vi "Inverse Kinematics Test.vi"() -> ()   [LabVIEW 2023]
uses:
  <vilib>/Analysis/coordinate.llb/Angle Units.ctl
  <vilib>/Analysis/coordinate.llb/Wrap Angle (scalar).vi
  <vilib>/Analysis/NI_AAL_Angle.lvlib
panel:
  in  "Turning Rate":dbl
  in  "Pod Max Turn Rate":dbl
  in  "stop":bool
  in  "Hide Components?":bool
  in  "dt":dbl
  in  "# Points":i32
  out "Expected Trajectory":cluster{dbl[], dbl[]}(graph)
  in  "Angular Velocity":dbl(slide) scale=-180.0..180.0
  out "Arcade Inputs":picture
  out "Visualization":cluster{dbl[], dbl[]}[](graph)
  in  "Radii":T1={"LF"=[-2.0, 2.0], "LB"=[-2.0, -2.0], "RF"=[2.0, 2.0], "RB"=[2.0, -2.0]} {"RB" format="%.2f"; "RF" format="%.2f"; "LB" format="%.2f"; "LF" format="%.2f"}
  # "Front (1)"
  # "Left (-1)"
  # "Right (1)"
  # "Back (-1)"
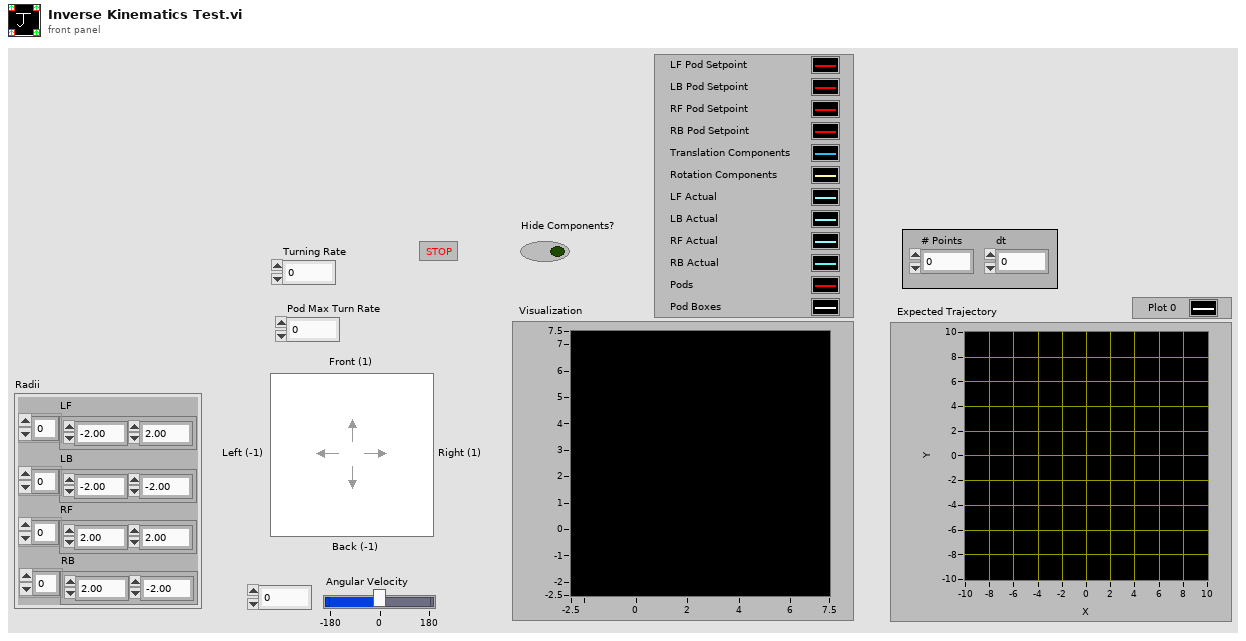
[diagram p1: front panel]
types:
  T1 = cluster{"LF":dbl[], "LB":dbl[], "RF":dbl[], "RB":dbl[]}
  T2 = cluster{"Plot.Plot Color":u32, "Plot.Line Style":u8}
  T3 = typedef "LVMouseTypeDef.ctl" = cluster{"Mouse Position":cluster{"X":i32, "Y":i32}, "Mouse Modifiers":cluster{"Button Down":bool, "Shift Mod":bool, "Menu Mod":bool, "Option Mod":bool}}
  T4 = typedef "LVBoundsTypeDef.ctl" = cluster{"Width":u32, "Height":u32}
  T5 = typedef "Pod Setpoints.ctl" = cluster{"Left Front":cluster{"Velocity":dbl, "Theta":dbl}, "Left Back":cluster{"Velocity":dbl, "Theta":dbl}, "Right Front":cluster{"Velocity":dbl, "Theta":dbl}, "Right Back":cluster{"Velocity":dbl, "Theta":dbl}}
  T6 = typedef "NI_AAL_Angle.lvlib/Angle Units.ctl" = i32
  T7 = cluster{"[0]":dbl, "[1]":dbl, "[2]":dbl, "[3]":dbl}
  T8 = cluster{"[0]":cluster{"Velocity":dbl, "Theta":dbl}, "[1]":cluster{"Velocity":dbl, "Theta":dbl}, "[2]":cluster{"Velocity":dbl, "Theta":dbl}, "[3]":cluster{"Velocity":dbl, "Theta":dbl}}
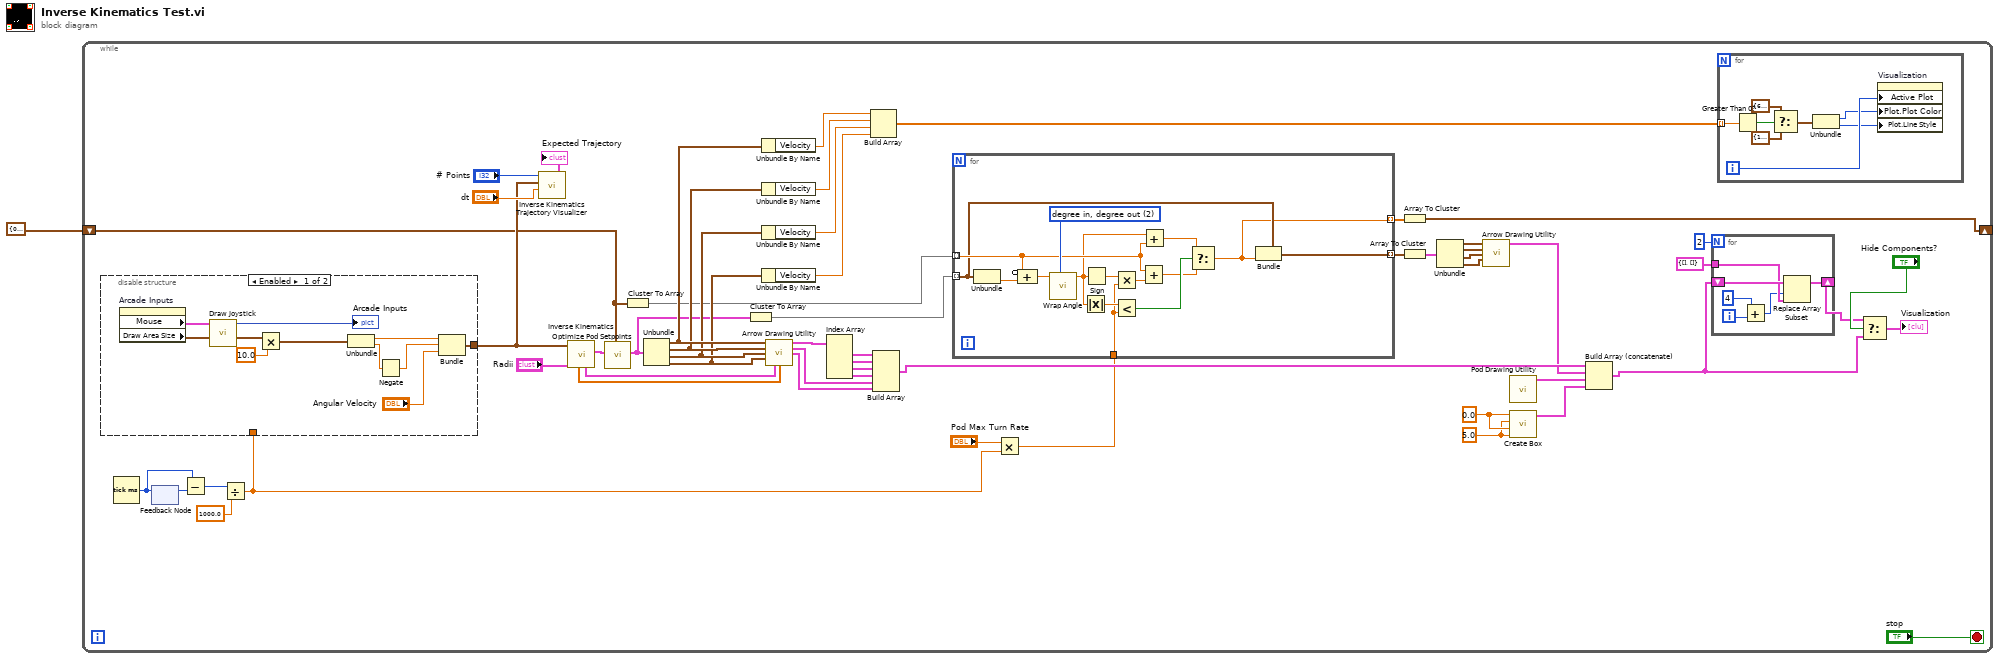
[diagram p0: block diagram]
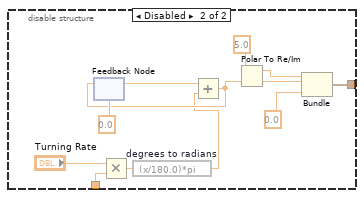
[diagram p2: hidden frame]
diagram:
  n1 = while {
    shift-right: [w20] -> _
    shift-left: cluster{"LF":dbl, "LB":dbl, "RF":dbl, "RB":dbl} {"LF"=0.0, "LB"=0.0, "RF"=0.0, "RB"=0.0} ("Current Pod Steering") -> [w25]
    stop <- "stop" stop-if-true
    w55 = 5.0 ("Right")
    w56 = 0.0 ("Left")
    n2 = Tick Count (ms)() -> (millisecond timer value=w7:u32)
    n3 = feedback-in #1(w7) -> ()
    n4 = feedback #1() -> (w8:u32)  [unwired: 1 in]
    n5 = Subtract(x=w7, y=w8) -> (x-y=w6:u32)
    n6 = Divide(x=w6, y=1000.0) -> (x/y=w4:dbl)
    n7 = disable-structure shown="Enabled" {
      disable-tunnel: [w73 w95] -> w32
      disable-tunnel: w4 -> [_ w92]
      frame Enabled {
        n8 = property on="Arcade Inputs" class="Pict"() -> ("Mouse"=w82:T3, "Draw Area Size"=w81:T4)  [unwired: 2 in, 2 out]
        n9 = call "Draw Joystick.vi"("Size"=w81, "Mouse"=w82) -> ("JS Coords"=w79:cluster{"X":dbl, "Y":dbl}, "Arcade Inputs"=→"Arcade Inputs":picture)  [unwired: 8 in]
        n10 = Multiply(x=w79, y=10.0 ("Angular Velocity")) -> (x*y=w78:cluster{"X":dbl, "Y":dbl})
        n11 = Unbundle(w78) -> ("X"=w76:dbl, "Y"=w80:dbl)
        n12 = Negate(x=w80) -> (-x=w75:dbl)
        n13 = Bundle("X"=w76, w75, "Angular Velocity"="Angular Velocity") -> (w73:cluster{"X":dbl, dbl, "Angular Velocity":dbl})  [unwired: 1 in]
      }
      frame Disabled {
        n14 = feedback #2(0.0) -> (w90:dbl)
        n15 = Multiply(x="Turning Rate", y=w92) -> (x*y=w85:dbl)
        n16 = expression code="(x/180.0)*pi" "degrees to radians"(w85) -> (w84:dbl)
        n17 = Add(x=w90, y=w84) -> (x+y=w89:dbl)
        n18 = feedback-in #2(w89) -> ()
        n19 = Polar To Re/Im(2:w89, 3:5.0 ("r")) -> (0:w86:dbl, 1:w87:dbl)
        n20 = Bundle(w87, w86, 0.0) -> (w95:cluster{dbl, dbl, dbl})  [unwired: 1 in]
      }
    }
    n21 = call "Inverse Kinematics Trajectory Visualizer.vi"("dt"="dt", "Target Velocity"=w32, "# Points"="# Points") -> ("Points"=→"Expected Trajectory":cluster{dbl[], dbl[]})  [unwired: 8 in]
    n22 = call "Inverse Kinematics.vi"("Radii (ft)"="Radii", "Target Velocity (ft/s and deg/s)"=w32) -> ("Pod Setpoints (ft/s and deg)"=w26:T5, "cross products"=w51:T1, "translation"=w50:dbl[])  [unwired: 7 in]
    n23 = call "Optimize Pod Setpoints.vi"("Current Pod Steering (deg)"=w25, "Initial Pod Setpoints (ft/s and deg)"=w26) -> ("Optimized Pod Setpoints (ft/s and deg)"=w23:T5)  [unwired: 9 in]
    n24 = Cluster To Array(cluster=w25) -> (array=w24:dbl[])
    n25 = Unbundle(w23) -> ("Left Front"=w30:cluster{"Velocity":dbl, "Theta":dbl}, "Left Back"=w29:cluster{"Velocity":dbl, "Theta":dbl}, "Right Front"=w28:cluster{"Velocity":dbl, "Theta":dbl}, "Right Back"=w27:cluster{"Velocity":dbl, "Theta":dbl})
    n26 = Cluster To Array(cluster=w23) -> (array=w22:cluster{"Velocity":dbl, "Theta":dbl}[])
    n27 = Unbundle By Name(w30) -> ("Velocity"=w37:dbl)
    n28 = Unbundle By Name(w29) -> ("Velocity"=w36:dbl)
    n29 = Unbundle By Name(w28) -> ("Velocity"=w35:dbl)
    n30 = Unbundle By Name(w27) -> ("Velocity"=w34:dbl)
    n31 = call "Arrow Drawing Utility.vi"("LF Pod Setpoint"=w30, "LB Pod Setpoint"=w29, "RF Pod Setpoint"=w28, "RB Pod Setpoint"=w27, "cross products"=w51, "Translation"=w50) -> ("Pod Vectors"=w45:cluster{dbl[], dbl[]}[], "Translation Vectors"=w49:cluster{dbl[], dbl[]}, "Rotation Vectors"=w48:cluster{dbl[], dbl[]})  [unwired: 7 in]
    n32 = Index Array(array=w45) -> (element #1=w44:cluster{dbl[], dbl[]}, element #2=w43:cluster{dbl[], dbl[]}, element #3=w42:cluster{dbl[], dbl[]}, element #4=w41:cluster{dbl[], dbl[]})  [unwired: 4 in]
    n33 = Build Array(w37, w36, w35, w34) -> (w33:dbl[])
    n34 = Build Array(w44, w43, w42, w41, w49, w48) -> (w18:cluster{dbl[], dbl[]}[])
    n35 = Multiply(x="Pod Max Turn Rate", y=w4) -> (x*y=w2:dbl)
    n36 = for {
      tunnel: w22 -> [w61] mode=indexing
      tunnel: w24 -> [w66] mode=indexing
      tunnel: [w60] -> w19 mode=indexing
      tunnel: [w59] -> w21 mode=indexing
      tunnel: w2 -> [w58]
      w70 = T6 2 items=["radian in, radian out", "radian in, degree out", "degree in, degree out", "degree in, radian out"] ("angle units")
      n37 = Unbundle(w61) -> ("Theta"=w72:dbl)  [unwired: 1 out]
      n38 = Compound Arithmetic op=ADD(invert w66, w72) -> (w71:dbl)
      n39 = call-poly <vilib>:"Wrap Angle.vi"("angle units"=w70, "angle in"=w71) -> ("angle out"=w65:dbl)  [unwired: 8 in, 1 out]
      n40 = Absolute Value(x=w65) -> (abs(x)=w69:dbl)
      n41 = Sign(1:w65) -> (0:w68:dbl)
      n42 = Multiply(x=w68, y=w58) -> (x*y=w67:dbl)
      n43 = Less?(x=w69, y=w58) -> (x < y?=w64:bool)
      n44 = Add(x=w66, y=w67) -> (x+y=w62:dbl)
      n45 = Add(x=w65, y=w66) -> (x+y=w63:dbl)
      n46 = Select(t=w63, s=w64, f=w62) -> (s? t:f=w59:dbl)
      n47 = Bundle(cluster=w61, "Theta"=w59) -> (w60:cluster{"Velocity":dbl, "Theta":dbl})  [unwired: 1 in]
    }
    n48 = Array To Cluster(array=w21) -> (cluster=w20:T7)
    n49 = Array To Cluster(array=w19) -> (cluster=w17:T8)
    n50 = Unbundle(w17) -> ("[0]"=w16:cluster{"Velocity":dbl, "Theta":dbl}, "[1]"=w15:cluster{"Velocity":dbl, "Theta":dbl}, "[2]"=w14:cluster{"Velocity":dbl, "Theta":dbl}, "[3]"=w13:cluster{"Velocity":dbl, "Theta":dbl})
    n51 = call "Arrow Drawing Utility.vi"("LF Pod Setpoint"=w16, "LB Pod Setpoint"=w15, "RF Pod Setpoint"=w14, "RB Pod Setpoint"=w13) -> ("Pod Vectors"=w12:cluster{dbl[], dbl[]}[])  [unwired: 9 in, 2 out]
    n52 = call "Pod Drawing Utility.vi"() -> ("Cluster"=w11:cluster{dbl[], dbl[]})  [unwired: 11 in]
    n53 = call "Create Box.vi"("Top"=w55, "Bottom"=w56, "Right"=w55, "Left"=w56) -> ("Box"=w10:cluster{dbl[], dbl[]})  [unwired: 5 in, 2 out]
    n54 = Build Array (concatenate)(w18, w12, w11, w10) -> (w9:cluster{dbl[], dbl[]}[])
    n55 = for {
      N: 2 -> [_]
      tunnel: cluster{dbl[], dbl[]} {[], []} ("new element/subarray") -> [w108]
      shift-right: [w107] -> w38
      shift-left: w9 -> [w109]
      i -> [w106]
      n56 = Add(x=4, y=w106) -> (x+y=w104:i32)
      n57 = Replace Array Subset(array=w109, new element=w108, index=w104) -> (w107:cluster{dbl[], dbl[]}[])
    }
    n58 = for {
      tunnel: w33 -> [w102] mode=indexing
      i -> [w103]
      n59 = Greater Than 0?(x=w102) -> (x > 0?=w101:bool)
      n60 = Select(t=T2 {"Plot.Plot Color"=6618880, "Plot.Line Style"=0}, s=w101, f=T2 {"Plot.Plot Color"=16711680, "Plot.Line Style"=2}) -> (s? t:f=w98:T2)
      n61 = Unbundle(w98) -> ("Plot.Plot Color"=w97:u32, "Plot.Line Style"=w96:u8)
      n62 = property on="Visualization" class="XYGraph (strict)"("Active Plot"=w103, "Plot.Plot Color"=w97, "Plot.Line Style"=w96) -> ()  [unwired: 2 in, 2 out]
    }
    n63 = Select(t=w38, s="Hide Components?", f=w9) -> (s? t:f=→"Visualization":cluster{dbl[], dbl[]}[])
  }
